vi "ADFX_Do_Make.vi"(8 "error in (no error)":errorcluster, 11 "Data in":T1) -> (0 "error out":errorcluster, 3 "Data out":T1)   [LabVIEW 2015]
doc: "Makes a folder with all files from control in the proper naming scheme for the FX board."
uses:
  controls/AFXP Data.ctl
  controls/AFCP Setup.ctl
  <vilib>/Utility/sysdir.llb/System Directory Type.ctl
  <userlib>/_OpenG.lib/file/file.llb/File Exists - Scalar__ogtk.vi
  <userlib>/_OpenG.lib/file/file.llb/Build Path - Traditional__ogtk.vi
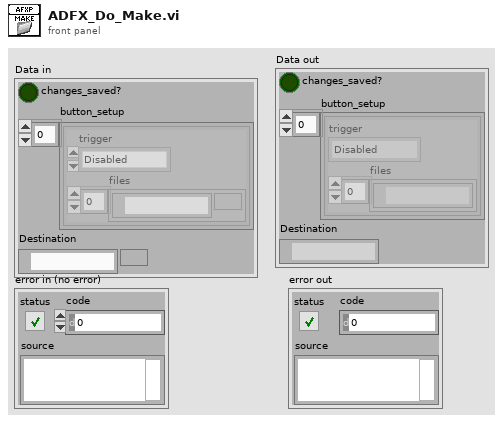
[diagram p1: front panel]
types:
  T1 = typedef "AFXP Data.ctl" = cluster{"changes_saved?":bool, "button_setup":T2[], "Destination":path}
  T2 = typedef "AFCP Setup.ctl" = cluster{"trigger":enum16{"Basic", "Hold-Loop", "Latch-Loop", "Next", "Random", "Disabled"}, "files":path[]}
  T3 = typedef "System Directory Type.ctl" = i32
  T4 = enum16{"Basic", "Hold-Loop", "Latch-Loop", "Next", "Random", "Disabled"}
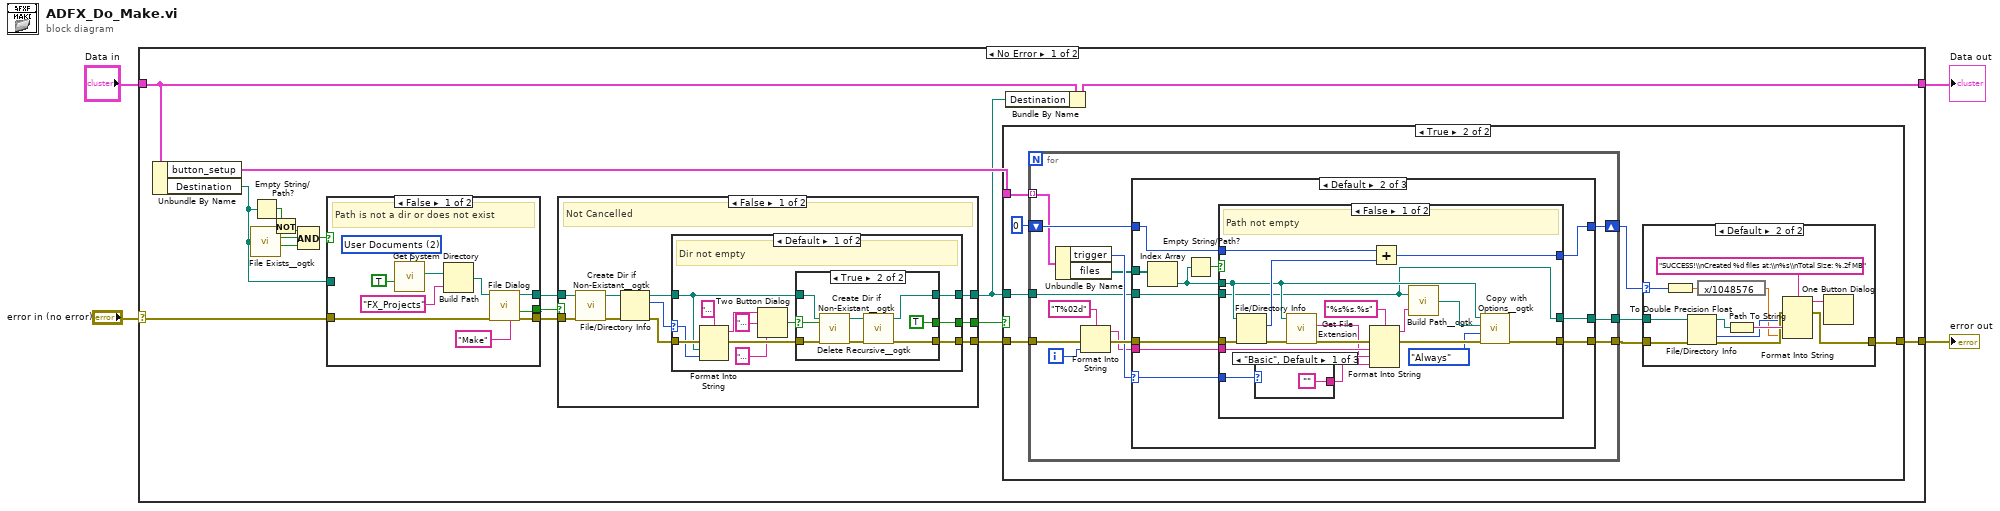
[diagram p0: block diagram]
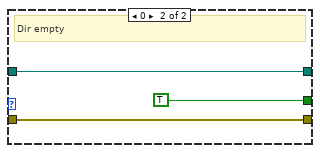
[diagram p3: hidden frame]
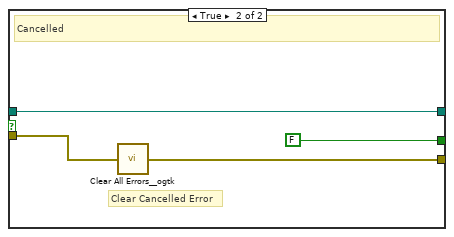
[diagram p4: hidden frame]
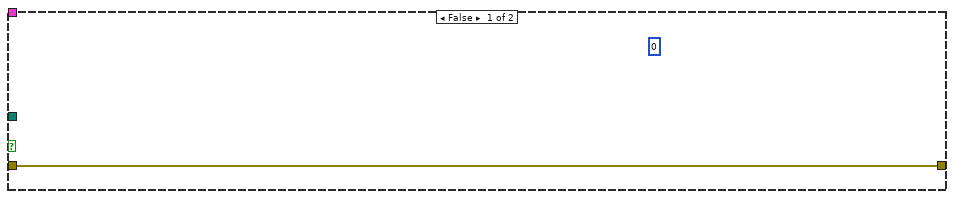
[diagram p5: hidden frame]
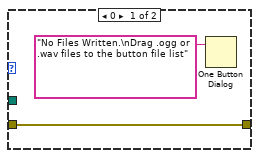
[diagram p6: hidden frame]
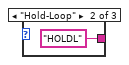
[diagram p8: hidden frame]
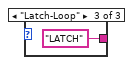
[diagram p9: hidden frame]
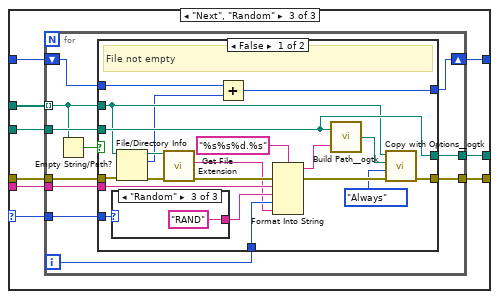
[diagram p11: hidden frame]
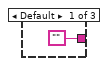
[diagram p12: hidden frame]
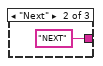
[diagram p13: hidden frame]
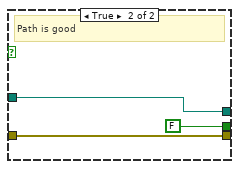
[diagram p15: hidden frame]
diagram:
  n1 = case shown="No Error" "error in (no error)" {
    selector: "error in (no error)" -> [w14 w196]
    tunnel: "Data in" -> [w13 w195]
    tunnel: [w19 w196] -> w1
    tunnel: [w8 w195] -> w2
    frame No Error {
      n2 = Unbundle By Name(w13) -> ("button_setup"=w20:T2[], "Destination"=w9:path)
      n3 = call-poly <userlib>:"File Exists__ogtk.vi"("file path"=w9) -> ("is directory"=w11:bool, "exists"=w10:bool)  [unwired: 6 in]
      n4 = Empty String/Path?(string/path=w9) -> (empty?=w12:bool)
      n5 = Not(x=w12) -> (.not. x?=w6:bool)
      n6 = Compound Arithmetic op=AND(w6, w11, w10) -> (w21:bool)
      n7 = case shown="False" w21 {
        tunnel: w14 -> [w191 w193]
        tunnel: w9 -> [_ w194]
        tunnel: [w190 w194] -> w15
        tunnel: [w189 w193] -> w17
        tunnel: [w187 FALSE ("cancelled")] -> w5
        frame False {
          w185 = T3 2 items=["User Home"=0, "User Desktop"=1, "User Documents"=2, "User Application Data"=3, "User Preferences"=4, "User Temporary"=5, "Public Documents"=6, "Public Application Data"=7, "Public Preferences"=8, "Public Cache"=13, "System Core Libraries"=9, "System Installed Libraries"=10, "Application Files"=11, "Boot Volume Root"=12] ("system directory type")
          # "Path is not a dir or does not exist"
          n8 = call <vilib>:"Get System Directory.vi"("create directory if not found? (F)"=TRUE, "system directory type"=w185) -> ("system directory"=w183:path)  [unwired: 9 in]
          n9 = Build Path(base path=w183, name or relative path="FX_Projects") -> (appended path=w182:path)
          n10 = call "File Dialog"("start path"=w182, "button label"="Make", "error in"=w191) -> ("selected path"=w190:path, "cancelled"=w187:bool, "error out"=w189:errorcluster)  [unwired: 9 in, 1 out]
        }
        frame True {
          # "Path is good"
        }
      }
      n11 = case shown="False" w5 {
        tunnel: [w30 FALSE ("T button?")] -> w18
        tunnel: w17 -> [w29 w59]
        tunnel: [w27 w58] -> w16
        tunnel: w15 -> [w25 w61]
        tunnel: [w23 w61] -> w7
        frame False {
          # "Not Cancelled"
          n12 = call <userlib>:"Create Dir if Non-Existant__ogtk.vi"("error in (no error)"=w29, "Directory Path"=w25) -> ("error out"=w26:errorcluster, "dup Directory Path"=w24:path)  [unwired: 7 in, 1 out]
          n13 = File/Directory Info(path=w24, error in=w26) -> (path out=w31:path, size=w22:i64, error out=w28:errorcluster)  [unwired: 4 out]
          n14 = case shown="Default" w22 {
            selector: w22 -> [w33 _]
            tunnel: w31 -> [w32 w57]
            tunnel: [w38 w57] -> w23
            tunnel: [w36 TRUE ("T button?")] -> w30
            tunnel: w28 -> [w43 w56]
            tunnel: [w37 w56] -> w27
            frame Default {
              # "Dir not empty"
              n15 = Format Into String(format string="WARNING: \"%s\" is not empty!\nAll %d files in this folder will be erased!" ("message"), error in=w43, w32, w33) -> (resulting string=w41:string, error out=w39:errorcluster)  [unwired: 1 in]
              n16 = Two Button Dialog(message=w41, 1:"ABORT" ("F button name (\"Cancel\")"), 2:"ERASE ALL" ("T button name (\"OK\")")) -> (T button?=w40:bool)
              n17 = case shown="True" w40 {
                selector: w40 -> [w44 w52]
                tunnel: w39 -> [w45 w54]
                tunnel: w32 -> [w46 w53]
                tunnel: [w46 w49] -> w38
                tunnel: [w45 w48] -> w37
                tunnel: [w44 TRUE] -> w36
                frame False {
                }
                frame True {
                  n18 = call <userlib>:"Delete Recursive__ogtk.vi"("error in (no error)"=w54, "Recursive? (FALSE)"=w52, "Path"=w53) -> ("error out"=w51:errorcluster, "dup Path"=w50:path)  [unwired: 7 in]
                  n19 = call <userlib>:"Create Dir if Non-Existant__ogtk.vi"("error in (no error)"=w51, "Directory Path"=w50) -> ("error out"=w48:errorcluster, "dup Directory Path"=w49:path)  [unwired: 7 in, 1 out]
                }
              }
            }
            frame 0 {
              # "Dir empty"
            }
          }
        }
        frame True {
          # "Clear Cancelled Error"
          # "Cancelled"
          n20 = call <userlib>:"Clear All Errors__ogtk.vi"("Error In"=w59) -> ("Error Out"=w58:errorcluster)  [unwired: 3 in]
        }
      }
      n21 = case shown="True" w18 {
        tunnel: w20 -> [_ w70]
        tunnel: w7 -> [_ w69]
        tunnel: w16 -> [w62 w68]
        tunnel: [w62 w65] -> w19
        frame False {
          (unwired) 0
        }
        frame True {
          n22 = for {
            tunnel: w70 -> [w94] mode=indexing
            tunnel: w69 -> [w89]
            tunnel: [w88] -> w66
            tunnel: w68 -> [w87]
            shift-right: [w86] -> w63
            shift-left: i64 0 -> [w97]
            tunnel: [w85] -> w64
            i -> [w91]
            n23 = Unbundle By Name(w94) -> ("trigger"=w95:T4, "files"=w93:path[])
            n24 = Format Into String(format string="T%02d", error in=w87, w91) -> (resulting string=w90:string, error out=w96:errorcluster)  [unwired: 1 in]
            n25 = case shown="Default" w95 {
              selector: w95 -> [_ w110 w143]
              tunnel: w93 -> [_ w111 w144]
              tunnel: w90 -> [_ w109 w142]
              tunnel: w89 -> [w98 w108 w140]
              tunnel: w96 -> [w100 w107 w139]
              tunnel: [w100 w106 w141] -> w88
              tunnel: w97 -> [w99 w102 w138]
              tunnel: [w99 w103 w137] -> w86
              tunnel: [w98 w101 w136] -> w85
              frame "Disabled" {
              }
              frame Default {
                n26 = Index Array(array=w111) -> (element=w105:path)  [unwired: 1 in]
                n27 = Empty String/Path?(string/path=w105) -> (empty?=w104:bool)
                n28 = case shown="False" w104 {
                  tunnel: w105 -> [w113 _]
                  tunnel: w110 -> [w127 _]
                  tunnel: w109 -> [w126 _]
                  tunnel: w108 -> [w112 w133]
                  tunnel: w107 -> [w114 w135]
                  tunnel: [w123 w135] -> w106
                  tunnel: [w116 w134] -> w103
                  tunnel: w102 -> [w118 w134]
                  tunnel: [w112 w133] -> w101
                  frame False {
                    # "Path not empty"
                    n29 = File/Directory Info(path=w113, error in=w114) -> (size=w117:i64, error out=w115:errorcluster)  [unwired: 5 out]
                    n30 = case shown="\"Basic\", Default" w127 {
                      tunnel: ["" "HOLDL" "LATCH"] -> w125
                      frame "Basic", Default {
                      }
                      frame "Hold-Loop" {
                      }
                      frame "Latch-Loop" {
                      }
                    }
                    n31 = call <vilib>:"Get File Extension.vi"("error in (no error)"=w115, "file"=w113) -> ("error out"=w121:errorcluster, "lowercase file extension"=w120:string)  [unwired: 5 in, 3 out]
                    n32 = Format Into String(format string="%s%s.%s", error in=w121, w126, w125, w120) -> (resulting string=w122:string, error out=w129:errorcluster)  [unwired: 1 in]
                    n33 = Add(x=w118, y=w117) -> (x+y=w116:i64)
                    n34 = call-poly <userlib>:"Build Path__ogtk.vi"("name or relative path"=w122, "base path"=w112) -> ("appended path"=w124:path)
                    n35 = call <userlib>:"Copy with Options__ogtk.vi"("error in (no error)"=w129, "Replace Mode (Never)"=enum16{"Never", "Always", "If Newer"}."Always", "target path"=w124, "source path"=w113) -> ("error out"=w123:errorcluster)  [unwired: 6 in, 1 out]
                  }
                  frame True {
                    # "Path Empty"
                  }
                }
              }
              frame "Next", "Random" {
                n36 = for {
                  tunnel: w144 -> [w150] mode=indexing
                  tunnel: w143 -> [w155]
                  tunnel: w142 -> [w154]
                  tunnel: [w153] -> w141
                  tunnel: w140 -> [w152]
                  tunnel: w139 -> [w151]
                  shift-right: [w147] -> w137
                  shift-left: w138 -> [w146]
                  tunnel: [w145] -> w136
                  i -> [w148]
                  n37 = Empty String/Path?(string/path=w150) -> (empty?=w149:bool)
                  n38 = case shown="False" w149 {
                    tunnel: w150 -> [w160 _]
                    tunnel: w155 -> [w172 _]
                    tunnel: w154 -> [w170 _]
                    tunnel: w148 -> [w164 _]
                    tunnel: [w168 w181] -> w153
                    tunnel: w152 -> [w175 w179]
                    tunnel: w151 -> [w161 w181]
                    tunnel: [w156 w180] -> w147
                    tunnel: w146 -> [w158 w180]
                    tunnel: [w175 w179] -> w145
                    frame False {
                      # "File not empty"
                      n39 = case shown="\"Random\"" w172 {
                        tunnel: ["" "NEXT" "RAND"] -> w169
                        frame Default {
                        }
                        frame "Next" {
                        }
                        frame "Random" {
                        }
                      }
                      n40 = File/Directory Info(path=w160, error in=w161) -> (path out=w159:path, size=w157:i64, error out=w162:errorcluster)  [unwired: 4 out]
                      n41 = call <vilib>:"Get File Extension.vi"("error in (no error)"=w162, "file"=w159) -> ("error out"=w165:errorcluster, "lowercase file extension"=w163:string)  [unwired: 5 in, 3 out]
                      n42 = Add(x=w158, y=w157) -> (x+y=w156:i64)
                      n43 = Format Into String(format string="%s%s%d.%s", error in=w165, w170, w169, w164, w163) -> (resulting string=w167:string, error out=w174:errorcluster)  [unwired: 1 in]
                      n44 = call-poly <userlib>:"Build Path__ogtk.vi"("name or relative path"=w167, "base path"=w175) -> ("appended path"=w166:path)
                      n45 = call <userlib>:"Copy with Options__ogtk.vi"("error in (no error)"=w174, "Replace Mode (Never)"=enum16{"Never", "Always", "If Newer"}."Always", "target path"=w166, "source path"=w160) -> ("error out"=w168:errorcluster)  [unwired: 6 in, 1 out]
                    }
                    frame True {
                      # "File Empty"
                    }
                  }
                }
              }
            }
          }
          n46 = case shown="Default" w63 {
            selector: w63 -> [_ w73]
            tunnel: w66 -> [w72 w76]
            tunnel: [w72 w75] -> w65
            tunnel: w64 -> [_ w74]
            frame 0 {
              n47 = One Button Dialog(message="No Files Written.\nDrag .ogg or .wav files to the button file list") -> ()  [unwired: 1 in, 1 out]
            }
            frame Default {
              n48 = To Double Precision Float(number=w73) -> (double precision float=w77:dbl)
              n49 = File/Directory Info(path=w74, error in=w76) -> (path out=w80:path, size=w79:i64, error out=w81:errorcluster)  [unwired: 4 out]
              n50 = expression code="x/1048576"(w77) -> (w78:dbl)
              n51 = Path To String(path=w80) -> (string=w83:string)
              n52 = Format Into String(format string="SUCCESS!\\nCreated %d files at:\\n%s\\nTotal Size: %.2f MB" ("message"), error in=w81, w79, w83, w78) -> (resulting string=w82:string, error out=w75:errorcluster)  [unwired: 1 in]
              n53 = One Button Dialog(message=w82) -> ()  [unwired: 1 in, 1 out]
            }
          }
        }
      }
      n54 = Bundle By Name(cluster=w13, "Destination"=w7) -> (w8:T1)
    }
    frame Error {
    }
  }
  "error out" <- w1
  "Data out" <- w2
